vi "board_fgv.vi"(7 "board actions (reset)":T1=enum."reset", 11 "move":string) -> (3 "board":picture[][](array[picture]))   [LabVIEW 2014]
doc: "Implement code in here to update board based on input <b>move</b>.\n\nTracks the current board using a functional global variable. Use <b>board actions</b> to indicate how to update the board and <b>move</b> to indicate where pieces are moving (i.e. using chess notation). Use <b>board action</b> \"reset\" once to initialize the chess pieces and start the board."
uses:
  board_actions.ctl
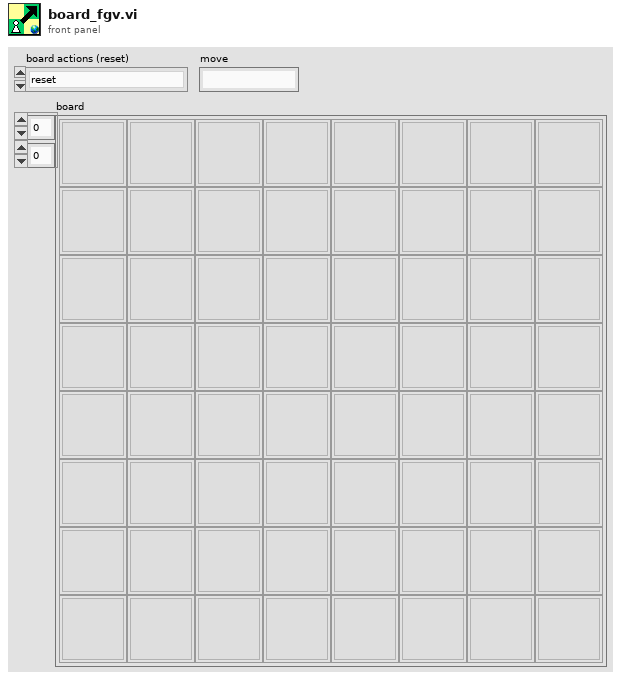
[diagram p1: front panel]
types:
  T1 = typedef "board_actions.ctl" = enum16{"move", "reset"}
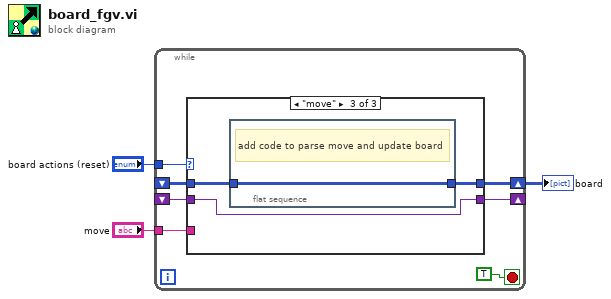
[diagram p0: block diagram]
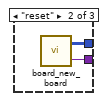
[diagram p3: hidden frame]
diagram:
  n1 = while {
    tunnel: "move" -> [w6]
    tunnel: "board actions (reset)" -> [w9]
    shift-right: [w8] -> w1
    shift-left: _ -> [w7]
    shift-right: [w5] -> _
    shift-left: _ -> [w4]
    stop <- TRUE stop-if-true
    n2 = case shown="\"move\"" w9 {
      tunnel: [w12 w14 w16] -> w8
      tunnel: w7 -> [w12 _ w17]
      tunnel: w6 -> [_ _ _]
      tunnel: [w11 w13 w15] -> w5
      tunnel: w4 -> [w11 _ w15]
      frame Default {
      }
      frame "reset" {
        n3 = call "board_new_board.vi"() -> ("chess pieces"=w13:variant, "new board"=w14:picture[][])  [unwired: 4 in]
      }
      frame "move" {
        n4 = flat-sequence {
          tunnel: w17 -> [w18]
          tunnel: [w18] -> w16
          frame #0 {
            # "add code to parse move and update board"
          }
        }
      }
    }
  }
  "board" <- w1
